vi "Send request (SubVI).vi"(3 "target":string, 4 "lockout_key":string, 6 "request content":string, 8 "error in (no error)":errorcluster, 9 "msgop":i32(ring) items=["0"=0, "1"=1, "6"=6, "7"=7, "8"=8, "9"=9], 10 "Channel in":refnum<class "Channel.lvclass">, 11 "Exchange.lvclass":refnum<class "Exchange.lvclass">) -> (1 "error IO":errorcluster, 2 "Array - String":string[](array[string]), 5 "timeout?":bool=TRUE)   [LabVIEW 2016]
uses:
  <vilib>/Distrio/LabbitMQ/Exchange/Exchange.lvclass
  <vilib>/Distrio/LabbitMQ/Channel/Channel.lvclass
  <vilib>/Distrio/LabbitMQ/Queue/Queue.lvclass
panel:
  in  "multi reply":bool
  in  "timeout":dbl=10.0 format="%#_13g"
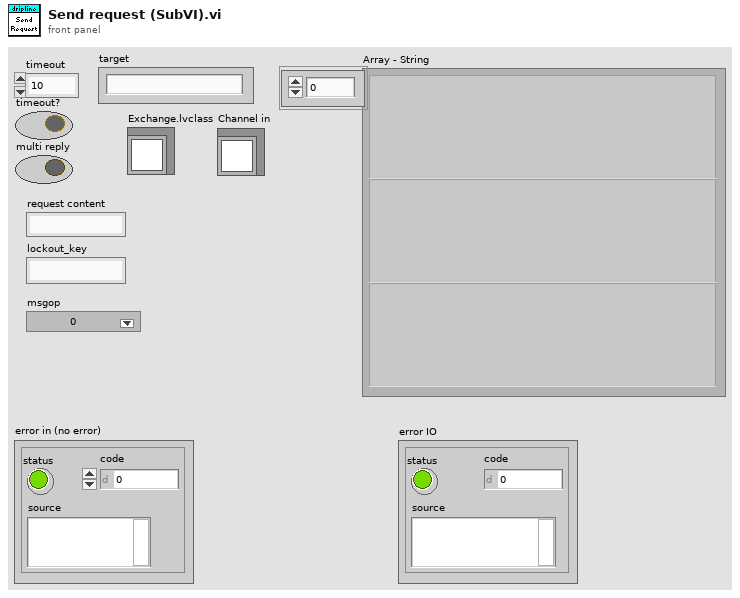
[diagram p1: front panel]
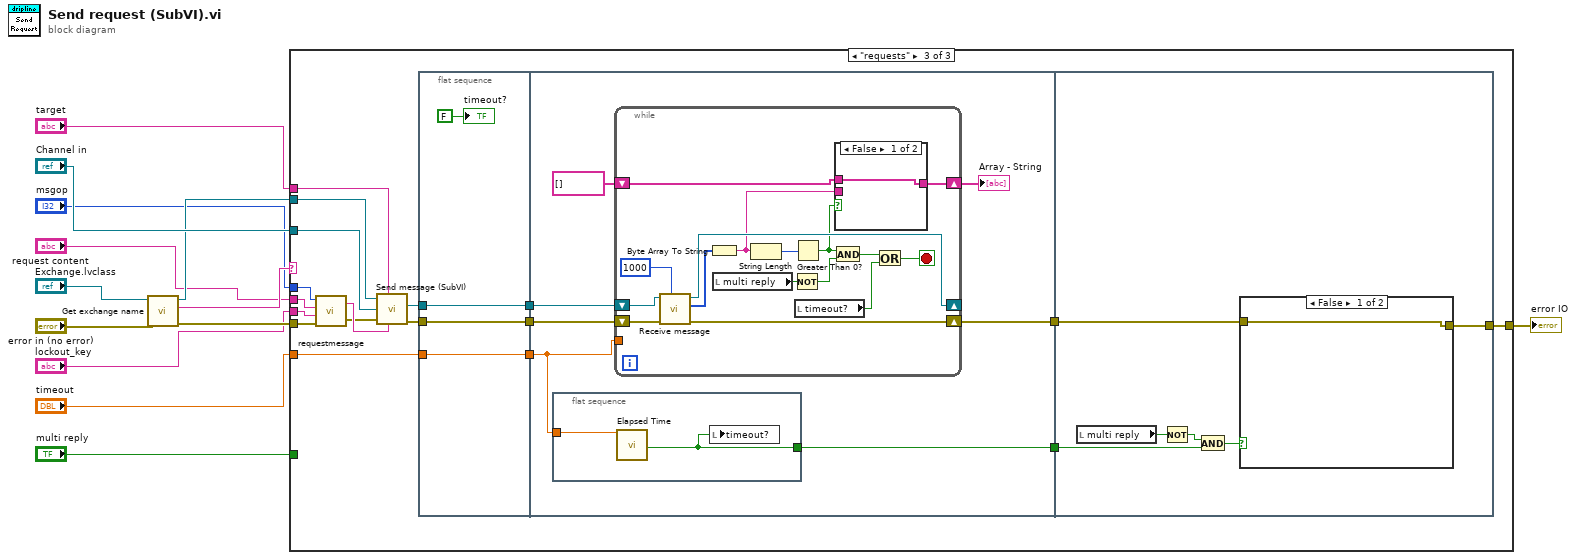
[diagram p0: block diagram]
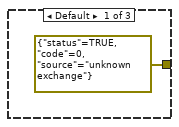
[diagram p2: hidden frame]
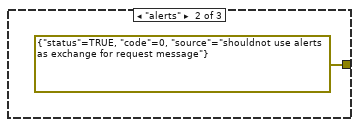
[diagram p3: hidden frame]
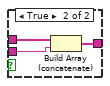
[diagram p4: hidden frame]
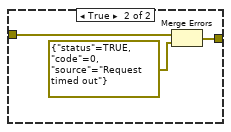
[diagram p5: hidden frame]
diagram:
  n1 = call <vilib>:"Get exchange name.vi"("error in (no error)"="error in (no error)", "Exchange in"="Exchange.lvclass") -> ("error out"=w12:errorcluster, "name"=w8:string, "Exchange out"=w10:refnum<class "Exchange.lvclass">)  [unwired: 7 in]
  n2 = case shown="\"requests\"" w8 {
    tunnel: "Channel in" -> [_ _ w33]
    tunnel: w12 -> [_ _ w29]
    tunnel: w10 -> [_ _ w32]
    tunnel: "target" -> [_ _ w31]
    tunnel: [errorcluster {"status"=TRUE, "code"=0, "source"="unknown exchange"} ("error constant") errorcluster {"status"=TRUE, "code"=0, "source"="shouldnot use alerts as exchange for request message"} ("error constant") w16] -> w3
    tunnel: "msgop" -> [_ _ w27]
    tunnel: "request content" -> [_ _ w26]
    tunnel: "lockout_key" -> [_ _ w25]
    tunnel: "timeout" -> [_ _ w24]
    tunnel: "multi reply" -> [_ _ _]
    frame Default {
    }
    frame "alerts" {
    }
    frame "requests" {
      n3 = call "requestmessage.vi"("error in (no error)"=w29, "lockout_key"=w25, "request content"=w26, "msgop"=w27) -> ("error out"=w28:errorcluster, "body"=w30:string)
      n4 = call "Send message (SubVI).vi"("Exchange.lvclass"=w32, "target"=w31, "Channel in"=w33, "error in (no error)"=w28, "body"=w30) -> ("Reply queue out"=w22:refnum<class "Queue.lvclass">, "error out"=w19:errorcluster)  [unwired: 2 out]
      n5 = flat-sequence {
        tunnel: w24 -> [w37]
        tunnel: [w37] -> w23
        tunnel: w22 -> [w35]
        tunnel: [w35] -> w21
        tunnel: [w34] -> w20
        tunnel: w19 -> [w34]
        tunnel: w23 -> [w44]
        tunnel: w21 -> [w43]
        tunnel: w20 -> [w42]
        tunnel: [w40] -> w18
        tunnel: [w39] -> w17
        tunnel: w18 -> [w69]
        tunnel: w17 -> [w72]
        tunnel: [w67] -> w16
        frame #0 {
          "timeout?" <- FALSE ("timeout?")
        }
        frame #1 {
          n6 = flat-sequence {
            tunnel: w44 -> [w46]
            tunnel: [w45] -> w40
            frame #0 {
              n7 = call "Elapsed Time"("Time Target (s)"=w46) -> ("Time has Elapsed"=w45:bool)  [unwired: 11 in, 7 out]
              n8 = local write "timeout?"(w45) -> ()
            }
          }
          n9 = while {
            tunnel: w44 -> [_]
            shift-right: [w60] -> _
            shift-left: w43 -> [w62]
            shift-right: [w59] -> w39
            shift-left: w42 -> [w61]
            shift-right: [w49] -> w38
            shift-left: string[] [] -> [w51]
            stop <- w53 stop-if-true
            n10 = call <vilib>:"Receive message.vi"("millisecondsTimeout"=1000, "error in (no error)"=w61, "Consumer in"=w62) -> ("error out"=w59:errorcluster, "message body"=w58:u8[], "Consumer out"=w60:refnum<class "Queue.lvclass">)  [unwired: 3 in, 3 out]
            n11 = Byte Array To String(unsigned byte array=w58) -> (string=w50:string)
            n12 = local read "multi reply"() -> (w48:bool)
            n13 = String Length(string=w50) -> (length=w56:i32)
            n14 = Not(x=w48) -> (.not. x?=w55:bool)
            n15 = Greater Than 0?(x=w56) -> (x > 0?=w52:bool)
            n16 = local read "timeout?"() -> (w57:bool)
            n17 = And(x=w52, y=w55) -> (x .and. y?=w54:bool)
            n18 = case shown="False" w52 {
              tunnel: w51 -> [w63 w66]
              tunnel: w50 -> [_ w65]
              tunnel: [w63 w64] -> w49
              frame False {
              }
              frame True {
                n19 = Build Array (concatenate)(w66, w65) -> (w64:string[])
              }
            }
            n20 = Or(x=w54, y=w57) -> (x .or. y?=w53:bool)
          }
          "Array - String" <- w38
        }
        frame #2 {
          n21 = local read "multi reply"() -> (w71:bool)
          n22 = Not(x=w71) -> (.not. x?=w70:bool)
          n23 = And(x=w70, y=w69) -> (x .and. y?=w68:bool)
          n24 = case shown="False" w68 {
            tunnel: w72 -> [w73 w76]
            tunnel: [w73 w74] -> w67
            frame False {
            }
            frame True {
              n25 = Merge Errors(w76, errorcluster {"status"=TRUE, "code"=0, "source"="Request timed out"} ("error constant")) -> (w74:errorcluster)
            }
          }
        }
      }
    }
  }
  "error IO" <- w3
